vi "generateWaveform.vi"(8 "error in (no error)":errorcluster, 11 "TrapezoidalWave in":refnum<class "TrapezoidalWave.lvclass">) -> (0 "error out":errorcluster, 2 "Signal Out":dbl, 3 "TrapezoidalWave out":refnum<class "TrapezoidalWave.lvclass">)   [LabVIEW 2015, in "TrapezoidalWave.lvclass"]
uses:
  TrapezoidalWave.lvclass
  TrapezoidalWave.lvclass/TrapezoidalWave.ctl
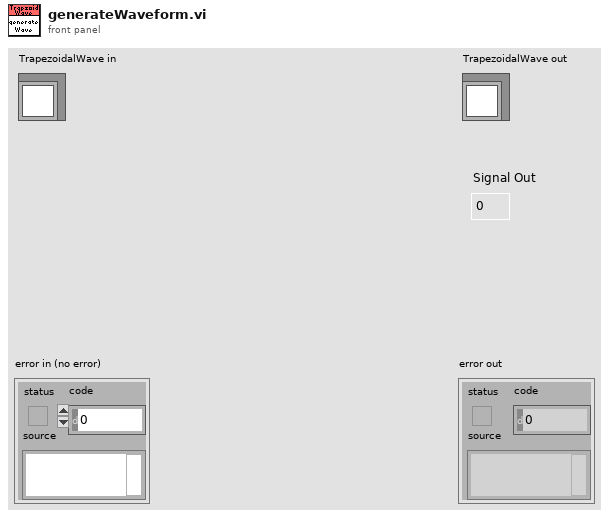
[diagram p1: front panel]
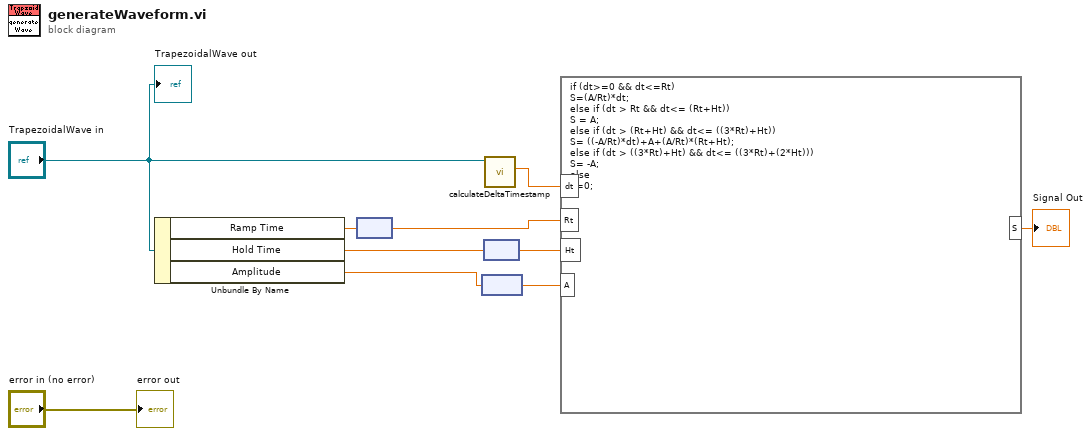
[diagram p0: block diagram]
diagram:
  n1 = Unbundle By Name("TrapezoidalWave in") -> ("Ramp Time"=w8:dbl[unit], "Hold Time"=w7:dbl[unit], "Amplitude"=w6:dbl[unit])
  n2 = node(w8) -> (w3:dbl)
  n3 = node(w6) -> (w5:dbl)
  n4 = node(w7) -> (w4:dbl)
  n5 = call "calculateDeltaTimestamp.vi"("TrapezoidalWave in"="TrapezoidalWave in") -> ("Delta Timestamp"=w9:dbl)  [unwired: 8 in, 2 out]
  n6 = formula code="if (dt>=0 && dt<=Rt)\nS=(A/Rt)*dt;\nelse if (dt > Rt && dt<= (Rt+Ht))\nS = A;\nelse if (dt > (Rt+Ht) && dt<= ((3*Rt)+Ht))\nS= ((-A/Rt)*dt)+A+(A/Rt)*(Rt+Ht);\nelse if (dt > ((3*Rt)+Ht) && dt<= ((3*Rt)+(2*Ht)))\nS= -A;\nelse \nS=0;"("dt"=w9, "Rt"=w3, "Ht"=w4, "A"=w5) -> ("S"=→"Signal Out":dbl)
  "error out" <- "error in (no error)"
  "TrapezoidalWave out" <- "TrapezoidalWave in"
